vi "Add Transition.vi"(0 "Tosca in":refnum<class "Parameters.lvclass">, 5 "Source":string, 7 "Target":string, 9 "Event":string, 11 "error in (no error)":errorcluster, 12 "Type":string) -> (4 "Tosca out":refnum<class "Parameters.lvclass">, 15 "error out":errorcluster)   [LabVIEW 2015, in "Parameters.lvclass"]
uses:
  Parameters.lvclass
  Parameters.lvclass/Parameters.ctl
  Typedefs/Tosca-Termination Condition Action.ctl
  State/State.lvclass/State.ctl
  State/Read TTL-only.vi
  State/State.lvclass
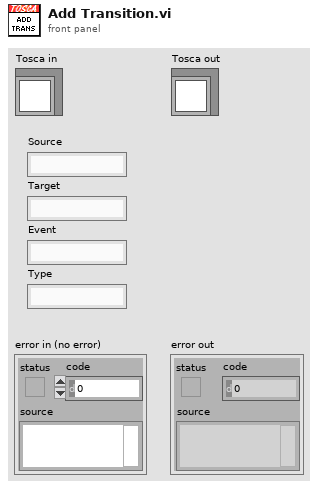
[diagram p1: front panel]
types:
  T1 = typedef "Tosca-Termination Condition Action.ctl" = enum16{"End state", "Complete state", "TTL only"}
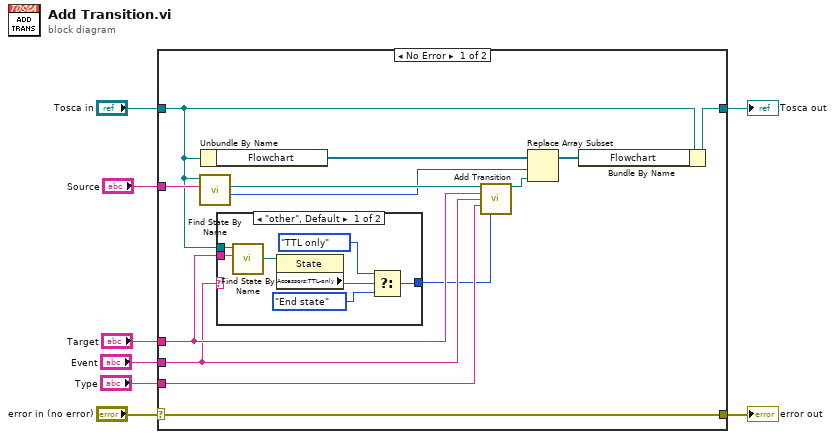
[diagram p0: block diagram]
diagram:
  n1 = case shown="No Error" "error in (no error)" {
    selector: "error in (no error)" -> [w21 w30]
    tunnel: [w21 w30] -> w7
    tunnel: [w17 w29] -> w5
    tunnel: "Tosca in" -> [w12 w29]
    tunnel: "Source" -> [w15 _]
    tunnel: "Target" -> [w11 _]
    tunnel: "Event" -> [w10 _]
    tunnel: "Type" -> [w19 _]
    frame No Error {
      n2 = call "Find State By Name.vi"("Name"=w15, "Tosca in"=w12) -> ("Index"=w13:i32, "State"=w14:refnum<class "State.lvclass">)  [unwired: 6 in, 2 out]
      n3 = Unbundle By Name(w12) -> ("Flowchart"=w20:refnum<class "State.lvclass">[])
      n4 = case shown="\"other\", Default" w10 {
        tunnel: w12 -> [w28 _]
        tunnel: w11 -> [w27 _]
        tunnel: [w23 _] -> w9
        frame "other", Default {
          n5 = call "Find State By Name.vi"("Name"=w27, "Tosca in"=w28) -> ("State"=w26:refnum<class "State.lvclass">)  [unwired: 6 in, 3 out]
          n6 = property class="State"(reference=w26) -> ("Accessors:TTL-only"=w25:bool)  [unwired: 1 in, 2 out]
          n7 = Select(t=Tosca-Termination_Condition_Action."TTL only", s=w25, f=Tosca-Termination_Condition_Action."End state" ("Action")) -> (s? t:f=w23:T1)
        }
        frame "Timeout" {
        }
      }
      n8 = call "Add Transition.vi"("State in"=w14, "Target"=w11, "Event"=w10, "Type"=w19, "Action"=w9) -> ("State out"=w18:refnum<class "State.lvclass">)  [unwired: 9 in, 1 out]
      n9 = Replace Array Subset(array=w20, new element=w18, index=w13) -> (w16:refnum<class "State.lvclass">[])
      n10 = Bundle By Name(cluster=w12, "Flowchart"=w16) -> (w17:refnum<class "Parameters.lvclass">)
    }
    frame Error {
    }
  }
  "error out" <- w7
  "Tosca out" <- w5
